vi "Lakeshore 336 Configure Channels.vi"(8 "error in":errorcluster, 10 "Ch Setup":T1[](array[typedef]) {"Heater Resistance (1:25 Ohms)" items=["25 Ohms"=1, "50 Ohms"=2]; "Max User Current (2.000)" format="%.3f"; "Heater Out Display (1:Current)" items=["Current"=1, "Power"=2]; "Max Current (0:User Specified)" items=["User Specified", "0.707 A", "1.0 A", "1.141 A", "2.0 A"]; "Mode (0:Off)" items=["Off", "Closed Loop PID", "Zone", "Open Loop"]; "Input (0:None)" items=["None", "A", "B", "C", "D"]}, 11 "VISA resource name":refnum<visa-resource-name>) -> (0 "error out":errorcluster, 3 "VISA resource name dup":refnum<visa-resource-name>)   [LabVIEW 2022 SP3, in "Lakeshore 336.lvclass"]
uses:
  Lakeshore 336.lvclass
  Lakeshore 336 Channel Settings cluster.ctl
  Lakeshore 336 PID cluster.ctl
  <instrlib>/lake_shore_336/Lake Shore 336/Lake Shore 336.lvlib
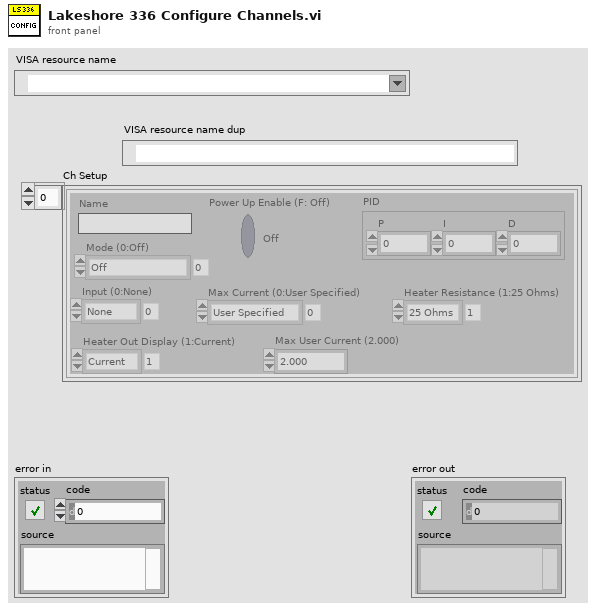
[diagram p1: front panel]
types:
  T1 = typedef "Lakeshore 336.lvclass/Lakeshore 336 Channel Settings cluster.ctl" = cluster{"Input (0:None)":u16, "Power Up Enable (F: Off)":bool, "Mode (0:Off)":u16, "Max Current (0:User Specified)":u16, "Heater Out Display (1:Current)":u16, "Max User Current (2.000)":dbl, "Heater Resistance (1:25 Ohms)":u16, "PID":T2, "Name":string}
  T2 = typedef "Lakeshore 336.lvclass/Lakeshore 336 PID cluster.ctl" = cluster{"P":dbl, "I":dbl, "D":dbl}
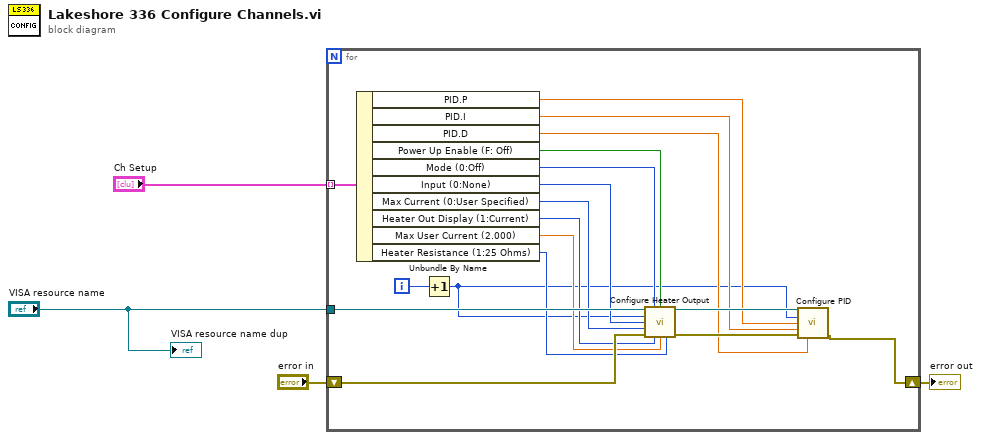
[diagram p0: block diagram]
diagram:
  n1 = for {
    tunnel: "VISA resource name" -> [w20]
    tunnel: "Ch Setup" -> [w19] mode=indexing
    shift-right: [w13] -> w2
    shift-left: "error in" -> [w14]
    i -> [w6]
    n2 = Unbundle By Name(w19) -> ("PID.P"=w7:dbl, "PID.I"=w8:dbl, "PID.D"=w9:dbl, "Power Up Enable (F: Off)"=w15:bool, "Mode (0:Off)"=w16:u16, "Input (0:None)"=w18:u16, "Max Current (0:User Specified)"=w17:u16, "Heater Out Display (1:Current)"=w12:u16, "Max User Current (2.000)"=w11:dbl, "Heater Resistance (1:25 Ohms)"=w10:u16)
    n3 = Increment(x=w6) -> (x+1=w5:i32)
    n4 = call <instrlib>:"Configure Heater Output.vi"("VISA resource name"=w20, "Mode (0:Off)"=w16, "Power Up Enable (F: Off)"=w15, "Heater Output (1:1)"=w5, "Input (0:None)"=w18, "Max Current (0:User Specified)"=w17, "error in (no error)"=w14, "Heater Out Display (1:Current)"=w12, "Max User Current (2.000)"=w11, "Heater Resistance (1:25 Ohms)"=w10) -> ("VISA resource name out"=w22:refnum<visa-resource-name>, "error out"=w21:errorcluster)  [unwired: 4 in]
    n5 = call <instrlib>:"Configure PID.vi"("VISA resource name"=w22, "Output's Control Loop (1:1)"=w5, "Gain (P) (50.0)"=w7, "Reset (I) (20.0)"=w8, "error in (no error)"=w21, "Rate (D) (0.0 %)"=w9) -> ("error out"=w13:errorcluster)  [unwired: 8 in, 1 out]
  }
  "error out" <- w2
  "VISA resource name dup" <- "VISA resource name"
